vi "Scan DQMH Modules EXEC.vi"(6 "TreeControl in":refnum<vi>, 7 "Data Cluster In":T2, 8 "error in":errorcluster, 11 "Scan DQMH Modules Argument":T1) -> (0 "error out":errorcluster, 5 "Data Cluster Out":T2={"DQMH Scan Results"={"All DQMH Modules Refs"=[], "All Modules Descriptions"=[], "All Modules type"=[], "Project References"={"Project Ref"=refnum, "Project Name"="", "Target"=refnum, "App Ref"=refnum}, "Dependencies"=[]}, "Current Selection"={"VI Ref"=refnum, "DQMH Lib Ref"=refnum}, "Module type"=enum."Singleton", "Module ID"=-1, "Theme"=FALSE, "Broadcast?"=FALSE, "Root Path"="", "Tree Selection"="", "Tree Map"={}})   [LabVIEW 2019, in "Panther Dashboard.lvlib"]
doc: "Gets the Singleton and Cloneable references and creates a list of each type of DQMH Modules"
uses:
  Panther Dashboard.lvlib
  Module Data--cluster.ctl
  DQMH Modules Info--cluster.ctl
  Module type--enum.ctl
  Project References--cluster.ctl
  <vilib>/National Instruments/Tree Map/Tree Map Data.ctl
  Scan DQMH Modules Argument--cluster.ctl
  <vilib>/National Instruments/Tree Map/API/List Roots.vi
  <vilib>/National Instruments/Tree Map/Utility/Into Tree Control Items.vi
  <vilib>/Delacor/Delacor QMH/Libraries/Scripting API/DQMH_Scripting API.lvlib
  <vilib>/National Instruments/Tree Map/Tree Map.lvlib
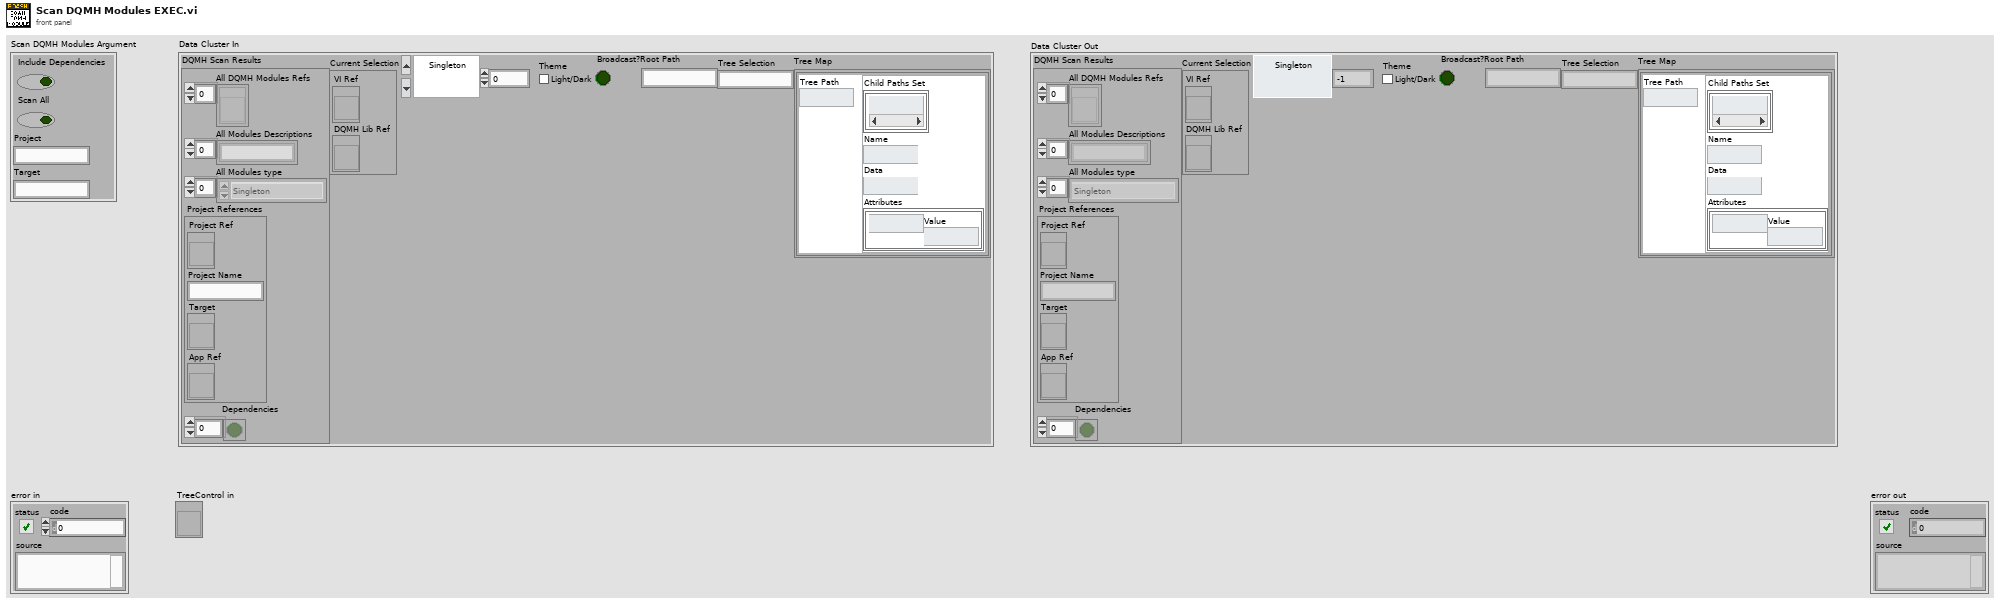
[diagram p1: front panel]
types:
  T1 = typedef "Panther Dashboard.lvlib/Scan DQMH Modules Argument--cluster.ctl" = cluster{"Include Dependencies":bool, "Scan All":bool, "Project":string, "Target":string}
  T2 = typedef "Panther Dashboard.lvlib/Module Data--cluster.ctl" = cluster{"DQMH Scan Results":T3, "Current Selection":cluster{"VI Ref":refnum<vi>, "DQMH Lib Ref":refnum<vi>}, "Module type":T4, "Module ID":i32, "Theme":bool, "Broadcast?":bool, "Root Path":string, "Tree Selection":string, "Tree Map":T6}
  T3 = typedef "Panther Dashboard.lvlib/DQMH Modules Info--cluster.ctl" = cluster{"All DQMH Modules Refs":refnum<vi>[], "All Modules Descriptions":string[], "All Modules type":T4[], "Project References":T5, "Dependencies":bool[]}
  T4 = typedef "Panther Dashboard.lvlib/Module type--enum.ctl" = enum16{"Singleton", "Cloneable"}
  T5 = typedef "Panther Dashboard.lvlib/Project References--cluster.ctl" = cluster{"Project Ref":refnum<vi>, "Project Name":string, "Target":refnum<vi>, "App Ref":refnum<vi>}
  T6 = typedef "Tree Map.lvlib/Tree Map Data.ctl" = map{string, cluster{"Child Paths Set":set{string}, "Name":string, "Data":string, "Attributes":map{string, string}}}
  T7 = typedef "DQMH_Scripting API.lvlib/Module Information--cluster.ctl" = cluster{"Library":refnum<vi>, "Qualified Name":string, "Path":path, "Cloneable":bool, "Under Dependencies":bool}
  T8 = cluster{"Left Cell String":string, "Child Text":string[], "Child Tag":string, "Item Indent":i32, "Child Only?":bool, "Glyph Index":i32}[]
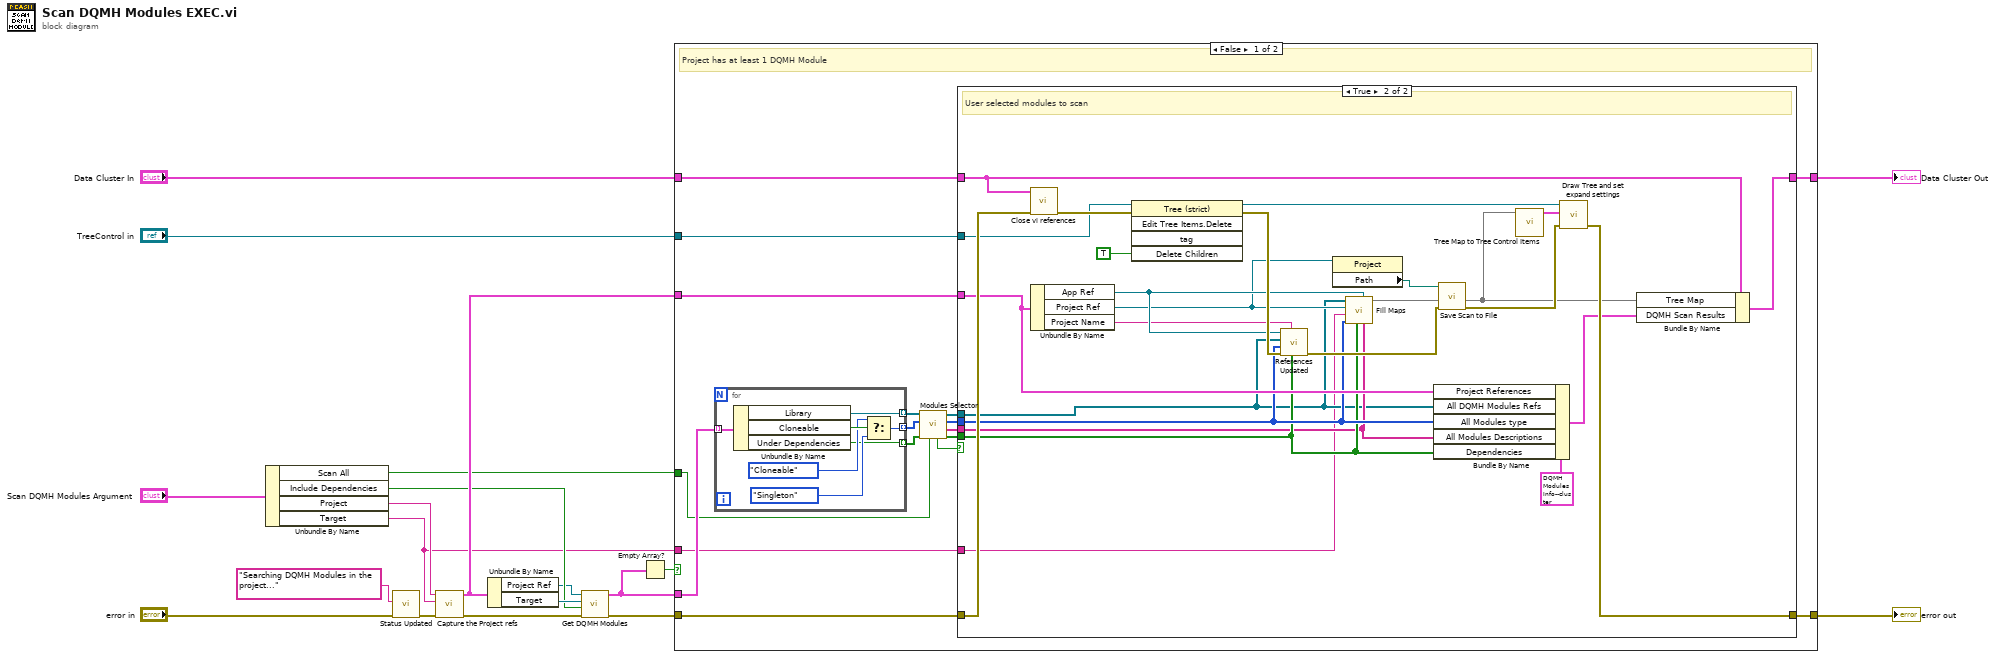
[diagram p0: block diagram]
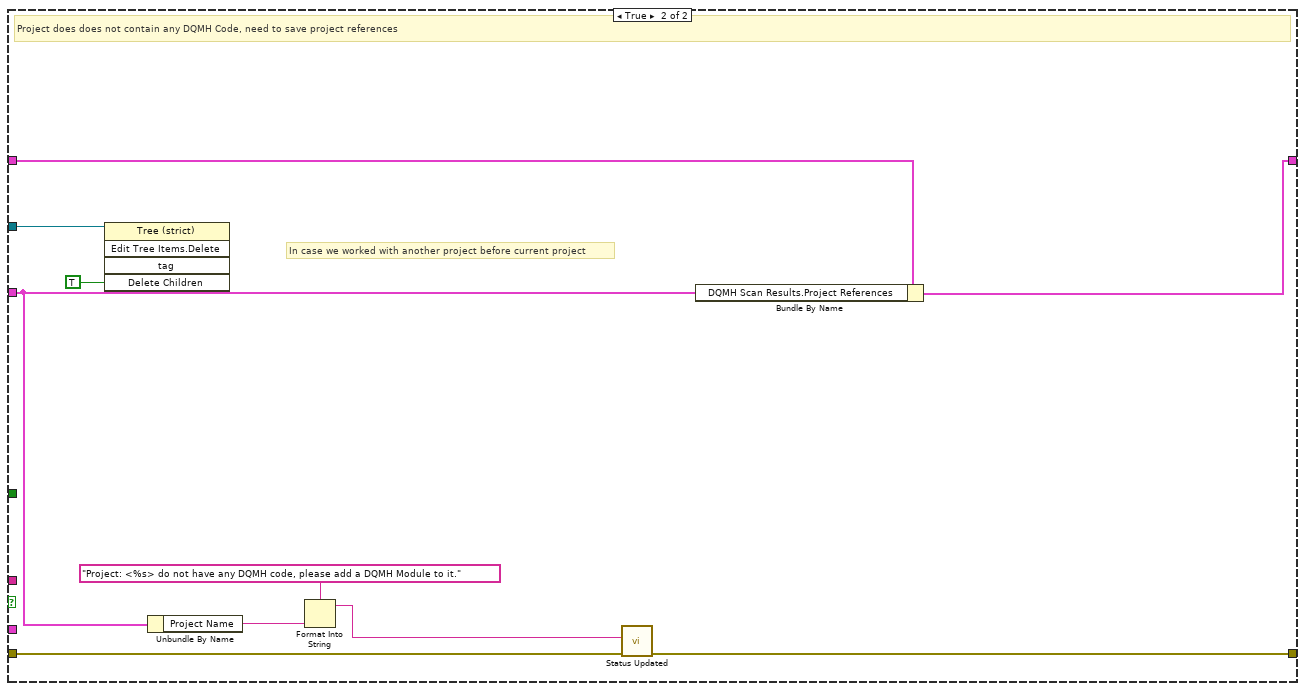
[diagram p3: hidden frame]
diagram:
  n1 = Unbundle By Name("Scan DQMH Modules Argument") -> ("Scan All"=w4:bool, "Include Dependencies"=w5:bool, "Project"=w3:string, "Target"=w1:string)
  n2 = call "Status Updated.vi"("error in (no error)"="error in", "Status"="Searching DQMH Modules in the project...") -> ("error out"=w16:errorcluster)  [unwired: 9 in]
  n3 = call "Capture the Project refs.vi"("error in"=w16, "Target Selection"=w1, "Project Selection"=w3) -> ("error out"=w17:errorcluster, "References"=w8:T5)  [unwired: 7 in]
  n4 = Unbundle By Name(w8) -> ("Project Ref"=w2:refnum<vi>, "Target"=w9:refnum<vi>)
  n5 = call <vilib>:"Get DQMH Modules.vi"("error in"=w17, "Include Dependencies (F)"=w5, "Target (My Computer)"=w9, "Project"=w2) -> ("error out"=w15:errorcluster, "DQMH Modules"=w6:T7[])  [unwired: 6 in]
  n6 = Empty Array?(array=w6) -> (empty?=w7:bool)
  n7 = case shown="False" w7 {
    tunnel: w15 -> [w36 w81]
    tunnel: [w35 w80] -> w18
    tunnel: w8 -> [w31 w77]
    tunnel: "Data Cluster In" -> [w29 w79]
    tunnel: [w28 w78] -> w13
    tunnel: "TreeControl in" -> [w26 w72]
    tunnel: w6 -> [w25 _]
    tunnel: w4 -> [w21 _]
    tunnel: w1 -> [w20 _]
    frame False {
      # "Project has at least 1 DQMH Module"
      n8 = for {
        tunnel: w25 -> [w71] mode=indexing
        tunnel: [w70] -> w24 mode=indexing
        tunnel: [w66] -> w23 mode=indexing
        tunnel: [w65] -> w22 mode=indexing
        n9 = Unbundle By Name(w71) -> ("Library"=w70:refnum<vi>, "Cloneable"=w68:bool, "Under Dependencies"=w65:bool)
        n10 = Select(t=Module_type--enum."Cloneable", s=w68, f=Module_type--enum."Singleton" ("Module type")) -> (s? t:f=w66:T4)
      }
      n11 = call "Modules Selector.vi"("Scan All"=w21, "Module In Dependencies?"=w22, "Modules Types In"=w23, "DQMH Modules In"=w24) -> ("Module In Dependencies?Out"=w30:bool[], "Descriptions"=w34:string[], "Modules Types Out"=w33:T4[], "DQMH Modules Out"=w32:refnum<vi>[], "Scan?"=w27:bool)  [unwired: 3 in]
      n12 = case shown="True" w27 {
        tunnel: w34 -> [_ w41]
        tunnel: w33 -> [_ w45]
        tunnel: w32 -> [_ w40]
        tunnel: w31 -> [_ w49]
        tunnel: w30 -> [_ w42]
        tunnel: w29 -> [w37 w54]
        tunnel: [w37 w55] -> w28
        tunnel: w26 -> [_ w52]
        tunnel: w36 -> [w38 w62]
        tunnel: [w38 w61] -> w35
        tunnel: w20 -> [_ w39]
        frame False {
          # "User Cancel Scan process, do not redraw tree and keep previous selection"
        }
        frame True {
          # "User selected modules to scan"
          n13 = call "Close vi references.vi"("error in"=w62, "Data Cluster"=w54) -> ("error out"=w64:errorcluster)  [unwired: 9 in]
          n14 = Unbundle By Name(w49) -> ("App Ref"=w57:refnum<vi>, "Project Ref"=w46:refnum<vi>, "Project Name"=w47:string)
          n15 = invoke class="Tree (strict)" method="Edit Tree Items.Delete"(reference=w52, error in=w64, "Delete Children"=TRUE ("Delete Children?")) -> (reference out=w50:refnum<vi>, error out=w63:errorcluster)  [unwired: 2 in, 3 out]
          n16 = call "References Updated.vi"("Dependencies"=w42, "Project Name"=w47, "error in"=w63, "Modules Types"=w45, "Modules"=w40, "Application Instance"=w57) -> ("error out"=w60:errorcluster)  [unwired: 5 in]
          n17 = property class="Project"(reference=w46) -> ("Path"=w48:path)  [unwired: 1 in, 2 out]
          n18 = call "Fill Maps.vi"("All Module Descriptions"=w41, "App Ref"=w57, "Dependencies"=w42, "Modules Types"=w45, "Target"=w39, "Project Ref"=w46, "DQMH Modules"=w40) -> ("Tree Map out"=w44:T6)  [unwired: 4 in]
          n19 = Bundle By Name(cluster=T3 {"All DQMH Modules Refs"=[], "All Modules Descriptions"=[], "All Modules type"=[], "Project References"={"Project Ref"=refnum, "Project Name"="", "Target"=refnum, "App Ref"=refnum}, "Dependencies"=[]} ("DQMH Scan Results"), "Project References"=w49, "All DQMH Modules Refs"=w40, "All Modules type"=w45, "All Modules Descriptions"=w41, "Dependencies"=w42) -> (w56:T3)
          n20 = call "Save Scan to File.vi"("error in"=w60, "Tree Map in"=w44, "Path"=w48) -> ("error out"=w59:errorcluster, "Tree Map Out"=w43:T6)  [unwired: 7 in]
          n21 = call <vilib>:"Tree Map to Tree Control Items.vi"("Tree Map In"=w43) -> ("Tree Control Items"=w53:T8)  [unwired: 10 in]
          n22 = call "Draw Tree and set expand settings.vi"("error in"=w59, "Tree Control Items"=w53, "TreeControl in"=w50) -> ("error out"=w61:errorcluster)  [unwired: 8 in]
          n23 = Bundle By Name(cluster=w54, "Tree Map"=w43, "DQMH Scan Results"=w56) -> (w55:T2)
        }
      }
    }
    frame True {
      # "In case we worked with another project before current project"
      # "Project does does not contain any DQMH Code, need to save project references"
      n24 = invoke class="Tree (strict)" method="Edit Tree Items.Delete"(reference=w72, "Delete Children"=TRUE ("Delete Children?")) -> ()  [unwired: 3 in, 5 out]
      n25 = Unbundle By Name(w77) -> ("Project Name"=w76:string)
      n26 = Format Into String(format string="Project: <%s> do not have any DQMH code, please add a DQMH Module to it.", w76) -> (resulting string=w75:string)  [unwired: 2 in, 1 out]
      n27 = call "Status Updated.vi"("error in (no error)"=w81, "Status"=w75) -> ("error out"=w80:errorcluster)  [unwired: 9 in]
      n28 = Bundle By Name(cluster=w79, "DQMH Scan Results.Project References"=w77) -> (w78:T2)
    }
  }
  "error out" <- w18
  "Data Cluster Out" <- w13
